vi "_Recursively List Included Files.vi"(6 "pattern":string[](array[string])=["*.md"], 8 "apply _ filter?(T)":bool=TRUE, 10 "Language Ring":string, 11 "dir":path[](array[path])) -> (2 "Common Path":path, 3 "Array":path[](array[path]))   [LabVIEW 2017, in "csmdoc.lvlib"]
uses:
  csmdoc.lvlib
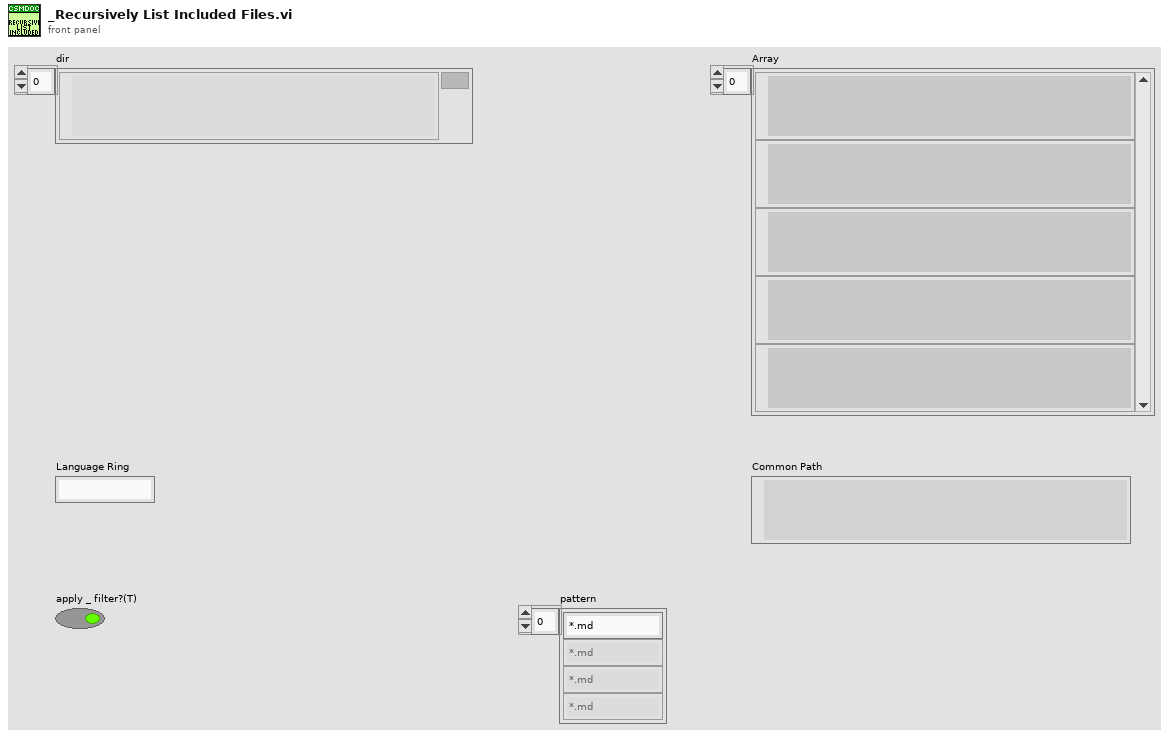
[diagram p1: front panel]
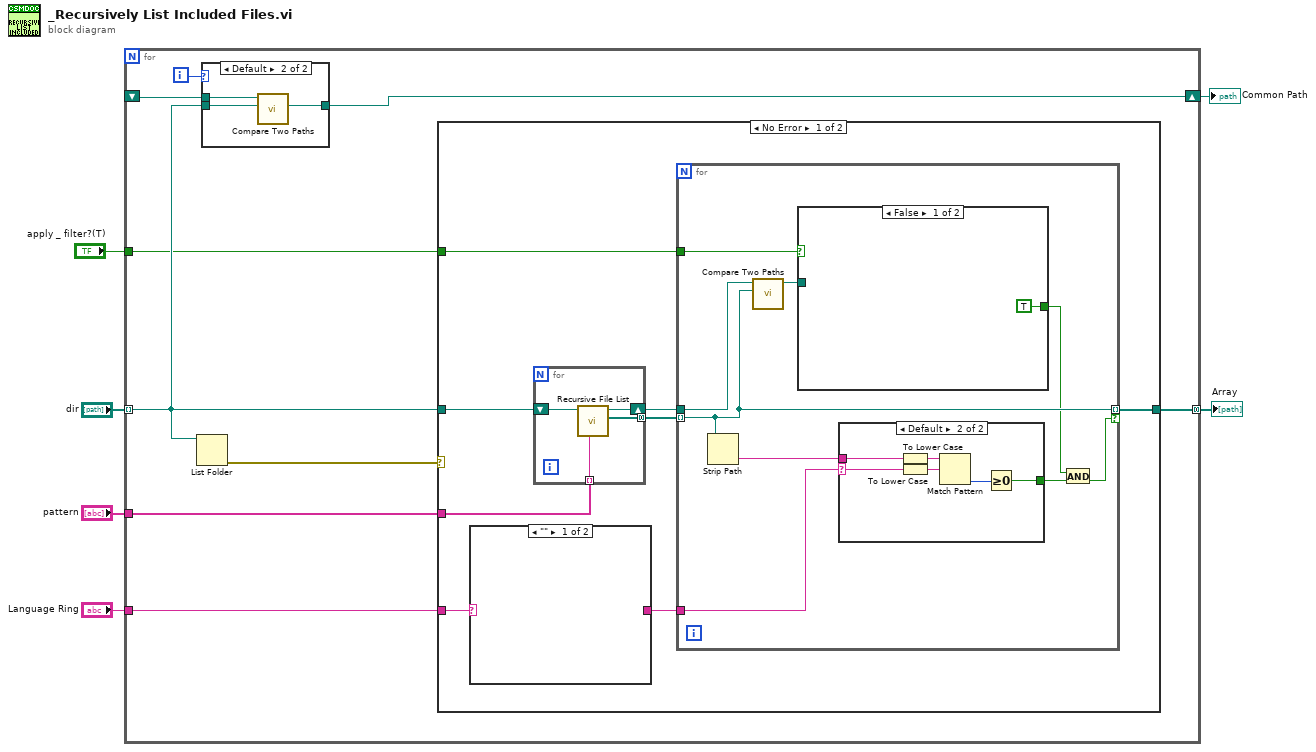
[diagram p0: block diagram]
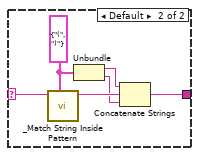
[diagram p2: hidden frame]
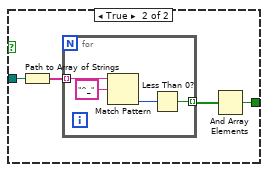
[diagram p3: hidden frame]
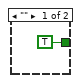
[diagram p4: hidden frame]
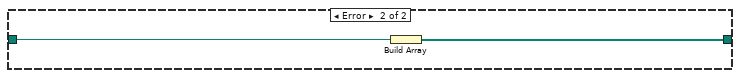
[diagram p5: hidden frame]
diagram:
  n1 = for {
    tunnel: "dir" -> [w11] mode=indexing
    tunnel: "Language Ring" -> [w15]
    tunnel: [w14] -> w6 mode=concatenating
    tunnel: "pattern" -> [w12]
    shift-right: [w10] -> w2
    shift-left: _ -> [w9]
    tunnel: "apply _ filter?(T)" -> [w7]
    i -> [w8]
    n2 = List Folder(path=w11) -> (error out=w13:errorcluster)  [unwired: 3 in, 3 out]
    n3 = case shown="Default" w8 {
      tunnel: [w61 w64] -> w10
      tunnel: w9 -> [_ w63]
      tunnel: w11 -> [w61 w62]
      frame 0 {
      }
      frame Default {
        n4 = call <vilib>:"Compare Two Paths.vi"("Path 2"=w62, "Path 1"=w63) -> ("Common Path"=w64:path)  [unwired: 6 in, 3 out]
      }
    }
    n5 = case shown="No Error" w13 {
      tunnel: w15 -> [w21 _]
      tunnel: [w20 w59] -> w14
      tunnel: w11 -> [w18 w60]
      tunnel: w12 -> [w17 _]
      tunnel: w7 -> [w16 _]
      frame No Error {
        n6 = case shown="\"\"" w21 {
          selector: w21 -> [_ w24]
          tunnel: [_ w25] -> w22
          frame "" {
          }
          frame Default {
            w29 = cluster{"left":string, "right":string} {"left"="(", "right"=")"} ("Cluster")
            n7 = call "_Match String Inside Pattern.vi"("Cluster"=w29, "string"=w24) -> ("String inside"=w28:string)  [unwired: 8 in, 1 out]
            n8 = Unbundle(w29) -> ("left"=w26:string, "right"=w27:string)
            n9 = Concatenate Strings(w26, w28, w27) -> (w25:string)
          }
        }
        n10 = for {
          tunnel: [w33] -> w23 mode=concatenating
          shift-right: [w32] -> w19
          shift-left: w18 -> [w31]
          tunnel: w17 -> [w30] mode=indexing
          n11 = call <vilib>:"Recursive File List.vi"("pattern"=w30, "Folder Path"=w31) -> ("All Files in Dir"=w33:path[], "dup Folder Path"=w32:path)  [unwired: 5 in, 3 out]
        }
        n12 = for {
          tunnel: w23 -> [w38] mode=indexing
          tunnel: [w38] -> w20 mode=indexing if=w36
          tunnel: w22 -> [w41]
          tunnel: w19 -> [w39]
          tunnel: w16 -> [w34]
          n13 = Strip Path(path=w38) -> (name=w42:string)  [unwired: 1 out]
          n14 = call <vilib>:"Compare Two Paths.vi"("Path 2"=w38, "Path 1"=w39) -> ("Relative Path from 1 to 2"=w37:path)  [unwired: 6 in, 3 out]
          n15 = case shown="False" w34 {
            tunnel: w37 -> [_ w47]
            tunnel: [TRUE w44] -> w35
            frame False {
            }
            frame True {
              n16 = Path to Array of Strings(0:w47) -> (2:w46:string[])  [unwired: 1 out]
              n17 = for {
                tunnel: w46 -> [w51] mode=indexing
                tunnel: [w48] -> w45 mode=indexing
                n18 = Match Pattern(string=w51, regular expression="^_") -> (offset past match=w49:i32)  [unwired: 1 in, 3 out]
                n19 = Less Than 0?(x=w49) -> (x < 0?=w48:bool)
              }
              n20 = And Array Elements(Boolean array=w45) -> (logical AND=w44:bool)
            }
          }
          n21 = case shown="Default" w41 {
            selector: w41 -> [_ w57]
            tunnel: w42 -> [_ w58]
            tunnel: [TRUE w55] -> w40
            frame "" {
            }
            frame Default {
              n22 = To Lower Case(string=w58) -> (all lower case string=w53:string)
              n23 = To Lower Case(string=w57) -> (all lower case string=w54:string)
              n24 = Match Pattern(string=w53, regular expression=w54) -> (offset past match=w56:i32)  [unwired: 1 in, 3 out]
              n25 = Greater Or Equal To 0?(x=w56) -> (x >= 0?=w55:bool)
            }
          }
          n26 = And(x=w35, y=w40) -> (x .and. y?=w36:bool)
        }
      }
      frame Error {
        n27 = Build Array(w60) -> (w59:path[])
      }
    }
  }
  "Array" <- w6
  "Common Path" <- w2
